vi "adjust_histogram_cursor.vi"(8 "error in (no error)":errorcluster, 10 "lock to bin edges":bool, 11 "histogram reference":refnum<vi>) -> (0 "error out":errorcluster)   [LabVIEW 2016]
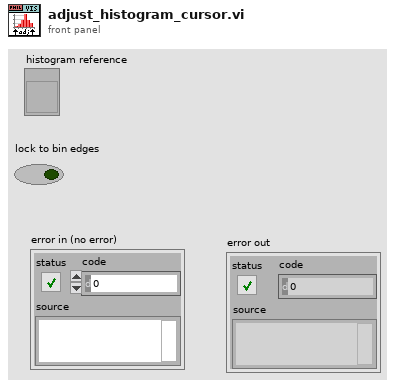
[diagram p1: front panel]
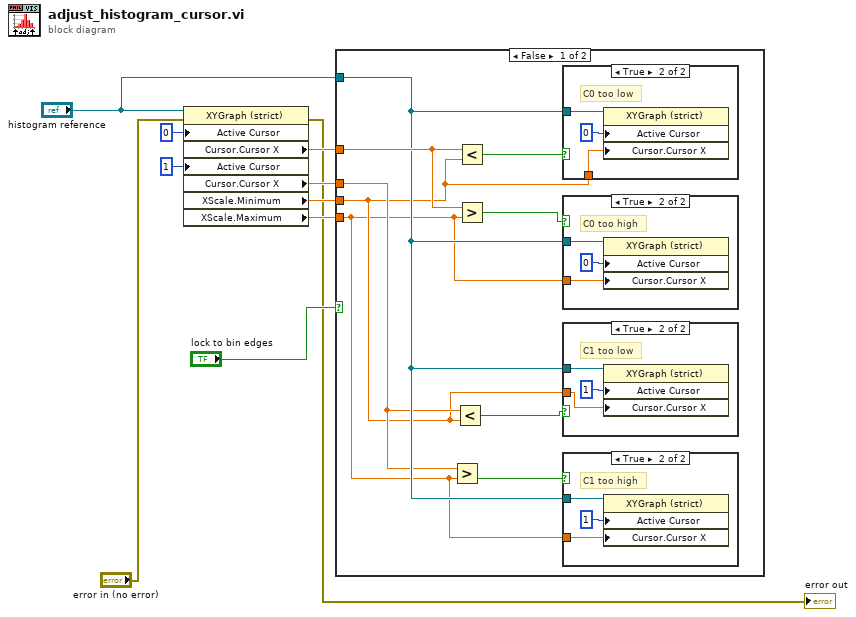
[diagram p0: block diagram]
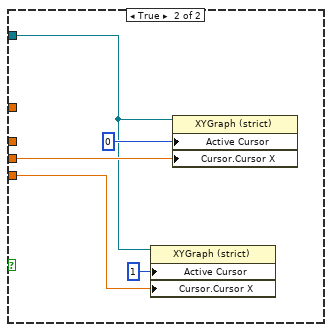
[diagram p6: hidden frame]
diagram:
  n1 = property on="Property Node" class="XYGraph (strict)"(reference="histogram reference", error in="error in (no error)", "Active Cursor"=0, "Active Cursor"=1) -> (error out=→"error out":errorcluster, "Cursor.Cursor X"=w8:dbl, "Cursor.Cursor X"=w6:dbl, "XScale.Minimum"=w5:dbl, "XScale.Maximum"=w4:dbl)  [unwired: 1 out]
  n2 = case shown="False" "lock to bin edges" {
    tunnel: w8 -> [w18 _]
    tunnel: "histogram reference" -> [w16 w32]
    tunnel: w6 -> [w13 _]
    tunnel: w5 -> [w12 w35]
    tunnel: w4 -> [w11 w33]
    frame False {
      n3 = Greater?(x=w13, y=w11) -> (0:w14:bool)
      n4 = Less?(x=w13, y=w12) -> (x < y?=w15:bool)
      n5 = Less?(x=w18, y=w12) -> (x < y?=w19:bool)
      n6 = Greater?(x=w18, y=w11) -> (0:w17:bool)
      n7 = case shown="True" w19 {
        tunnel: w16 -> [_ w30]
        tunnel: w12 -> [_ w29]
        frame False {
        }
        frame True {
          # "C0 too low"
          n8 = property on="Property Node" class="XYGraph (strict)"(reference=w30, "Active Cursor"=0, "Cursor.Cursor X"=w29) -> ()  [unwired: 1 in, 2 out]
        }
      }
      n9 = case shown="True" w17 {
        tunnel: w16 -> [_ w27]
        tunnel: w11 -> [_ w26]
        frame False {
        }
        frame True {
          # "C0 too high"
          n10 = property on="Property Node" class="XYGraph (strict)"(reference=w27, "Active Cursor"=0, "Cursor.Cursor X"=w26) -> ()  [unwired: 1 in, 2 out]
        }
      }
      n11 = case shown="True" w15 {
        tunnel: w16 -> [_ w24]
        tunnel: w12 -> [_ w23]
        frame False {
        }
        frame True {
          # "C1 too low"
          n12 = property on="Property Node" class="XYGraph (strict)"(reference=w24, "Active Cursor"=1, "Cursor.Cursor X"=w23) -> ()  [unwired: 1 in, 2 out]
        }
      }
      n13 = case shown="True" w14 {
        tunnel: w16 -> [_ w21]
        tunnel: w11 -> [_ w20]
        frame False {
        }
        frame True {
          # "C1 too high"
          n14 = property on="Property Node" class="XYGraph (strict)"(reference=w21, "Active Cursor"=1, "Cursor.Cursor X"=w20) -> ()  [unwired: 1 in, 2 out]
        }
      }
    }
    frame True {
      n15 = property on="Property Node" class="XYGraph (strict)"(reference=w32, "Active Cursor"=1, "Cursor.Cursor X"=w33) -> ()  [unwired: 1 in, 2 out]
      n16 = property on="Property Node" class="XYGraph (strict)"(reference=w32, "Active Cursor"=0, "Cursor.Cursor X"=w35) -> ()  [unwired: 1 in, 2 out]
    }
  }
